vi "Solenoid Control.vi"(2 "Defense Get":T1, 3 "Ball Get":T1, 4 "Both Down":bool, 5 "Both Up":bool, 6 "Ball Down":bool, 7 "Ball Up":bool) -> (0 "Defense Output":T1, 1 "Ball Output":T1)   [LabVIEW 2015]
uses:
  <vilib>/Rock Robotics/WPI/Solenoid/WPI_SolenoidValue.ctl
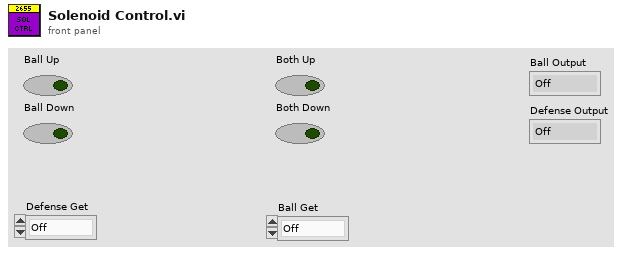
[diagram p1: front panel]
types:
  T1 = typedef "WPI_SolenoidValue.ctl" = enum16{"Off", "On", "Forward", "Reverse"}
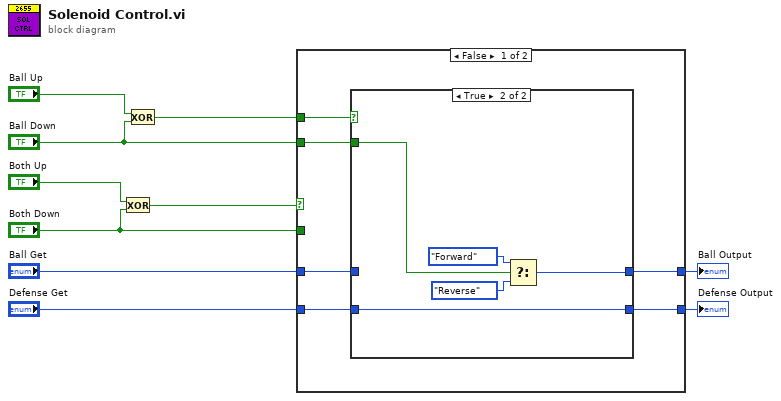
[diagram p0: block diagram]
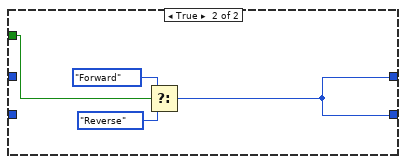
[diagram p3: hidden frame]
diagram:
  n1 = Exclusive Or(1:"Both Down", 2:"Both Up") -> (0:w9:bool)
  n2 = Exclusive Or(1:"Ball Down", 2:"Ball Up") -> (0:w6:bool)
  n3 = case shown="False" w9 {
    tunnel: [w15 w24] -> w2
    tunnel: "Both Down" -> [_ w27]
    tunnel: w6 -> [w16 _]
    tunnel: "Ball Down" -> [w14 _]
    tunnel: [w11 w24] -> w1
    tunnel: "Ball Get" -> [w13 _]
    tunnel: "Defense Get" -> [w12 _]
    frame False {
      n4 = case shown="True" w16 {
        tunnel: [w18 w22] -> w15
        tunnel: w14 -> [_ w23]
        tunnel: w13 -> [w18 _]
        tunnel: w12 -> [w17 w19]
        tunnel: [w17 w19] -> w11
        frame False {
        }
        frame True {
          n5 = Select(t=WPI_SolenoidValue."Forward", s=w23, f=WPI_SolenoidValue."Reverse" ("t")) -> (s? t:f=w22:T1)
        }
      }
    }
    frame True {
      n6 = Select(t=WPI_SolenoidValue."Forward", s=w27, f=WPI_SolenoidValue."Reverse" ("t")) -> (s? t:f=w24:T1)
    }
  }
  "Ball Output" <- w2
  "Defense Output" <- w1
